vi "Spartan CONFIG Global.vi"() -> ()   [LabVIEW 2011]
uses:
  ITK EXT/utils/keyedarr.llb/Keyed Array.ctl
panel:
  out "CONFIG":T1
  # "This control must not be on spartan version global\nupdater will fail"
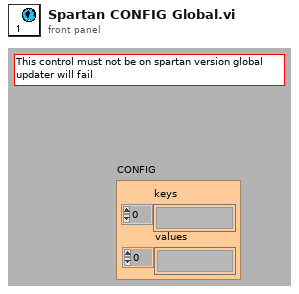
[diagram p1: front panel]
types:
  T1 = typedef "Keyed Array.ctl" = cluster{"keys":string[], "values":string[]}
diagram:
